vi "DC_Handler.vi"(9 "file":path, 11 "Operation":enum16{"Init", "Set"}(ring)) -> (1 "Event Registration Refnum":refnum<event-registration>)   [LabVIEW 2013, in "double click.lvlib"]
uses:
  double click.lvlib
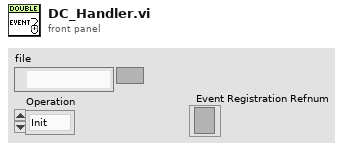
[diagram p1: front panel]
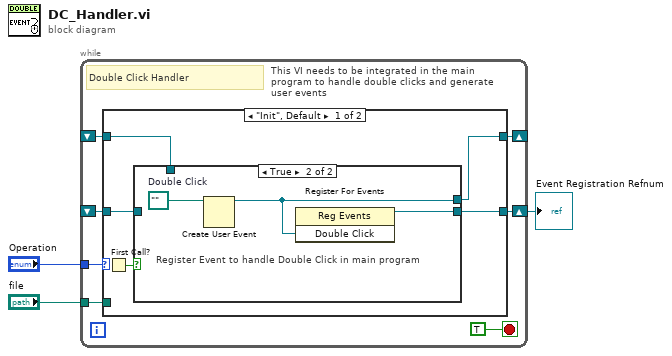
[diagram p0: block diagram]
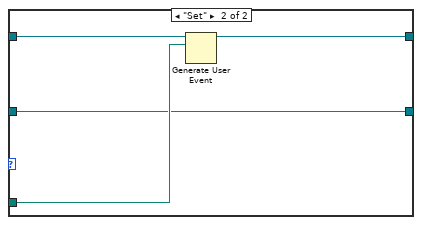
[diagram p3: hidden frame]
diagram:
  n1 = while {
    tunnel: "Operation" -> [w9]
    shift-right: [w8] -> _
    shift-left: _ -> [w7]
    tunnel: "file" -> [w6]
    shift-right: [w5] -> w1
    shift-left: _ -> [w4]
    stop <- TRUE stop-if-true
    # "This VI needs to be integrated in the main \nprogram to handle double clicks and generate\nuser events"
    # "Double Click Handler"
    n2 = case shown="\"Init\", Default" w9 {
      tunnel: [w15 w23] -> w8
      tunnel: w7 -> [w13 w24]
      tunnel: w6 -> [_ w22]
      tunnel: [w12 w21] -> w5
      tunnel: w4 -> [w11 w21]
      frame "Init", Default {
        n3 = First Call?() -> (First Call?: T/F=w14:bool)
        n4 = case shown="True" w14 {
          tunnel: [w17 w20] -> w15
          tunnel: w13 -> [w17 _]
          tunnel: [w16 w19] -> w12
          tunnel: w11 -> [w16 _]
          frame False {
          }
          frame True {
            w18 = path ""  # Double Click
            # "Register Event to handle Double Click in main program"
            n5 = Create User Event(user event datatype=w18) -> (user event=w20:refnum<user-event>)  [unwired: 1 in, 1 out]
            n6 = register-events(w20) -> (reference out=w19:refnum<event-registration>)  [unwired: 2 in, 1 out]
          }
        }
      }
      frame "Set" {
        n7 = Generate User Event(user event=w24, event data cluster=w22) -> (user event out=w23:refnum<user-event>)  [unwired: 2 in, 1 out]
      }
    }
  }
  "Event Registration Refnum" <- w1
